vi "Double Click Action Data.vi"(7 "Row":i32, 8 "Action List":T2(array[cluster])=[{"Action Name"="Enable Motor", "JSON info"=[{"path"="Index", "data type"=enum."INT"}], "String Format"="%(Action Name) %(Index)"}, {"Action Name"="Disable Motor", "JSON info"=[{"path"="Index", "data type"=enum."INT"}], "String Format"="%(Action Name) %(Index)"}, {"Action Name"="Move Motor", "JSON info"=[{"path"="Index", "data type"=enum."INT"}, {"path"="Destination", "data type"=enum."DBL"}], "String Format"="%(Action Name) %(Index) to %(Destination)"}], 9 "Array of Data Types in":T1(array[cluster]), 10 "Array of Data Names&Defaults in":cluster{"Data Names&Defaults":string[][]}[](array[cluster]), 11 "MCListbox Ref":refnum<vi>) -> (1 "Array of Data Types out":T1(array[cluster]), 2 "Array of Data Names&Defaults out":cluster{"Data Names&Defaults":string[][]}[](array[cluster]))   [LabVIEW 2016, in "Hardware.lvlib" / "Motions.lvlib" / "Motions.lvclass"]
uses:
  <userlib>/Common Components/Hardware/Abstract System/Motions/Motions/Motions.lvclass
  <userlib>/TSPopup/TSPopup.lvlib
panel:
  in  "Motor Labels":string[](array[string])
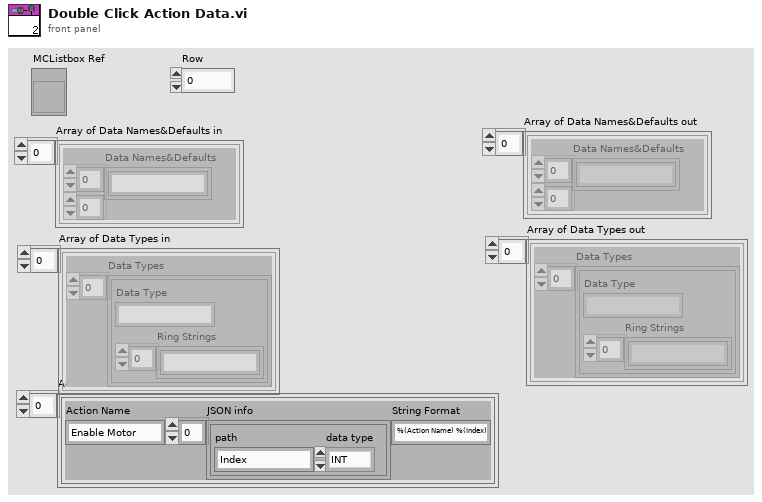
[diagram p1: front panel]
types:
  T1 = cluster{"Data Types":cluster{"Data Type":string, "Ring Strings":string[]}[]}[]
  T2 = cluster{"Action Name":string, "JSON info":cluster{"path":string, "data type":enum16{"INT", "DBL", "BOOL", "String"}}[], "String Format":string}[]
  T3 = cluster{"Data Type":string, "Captioned/Ring Strings":string[]}
  T4 = cluster{"path":string, "data type":enum16{"INT", "DBL", "BOOL", "String"}}[]
  T5 = cluster{"Data Types":cluster{"Data Type":string, "Ring Strings":string[]}[]}
  T6 = cluster{"Data Type":string, "Ring Strings":string[]}[]
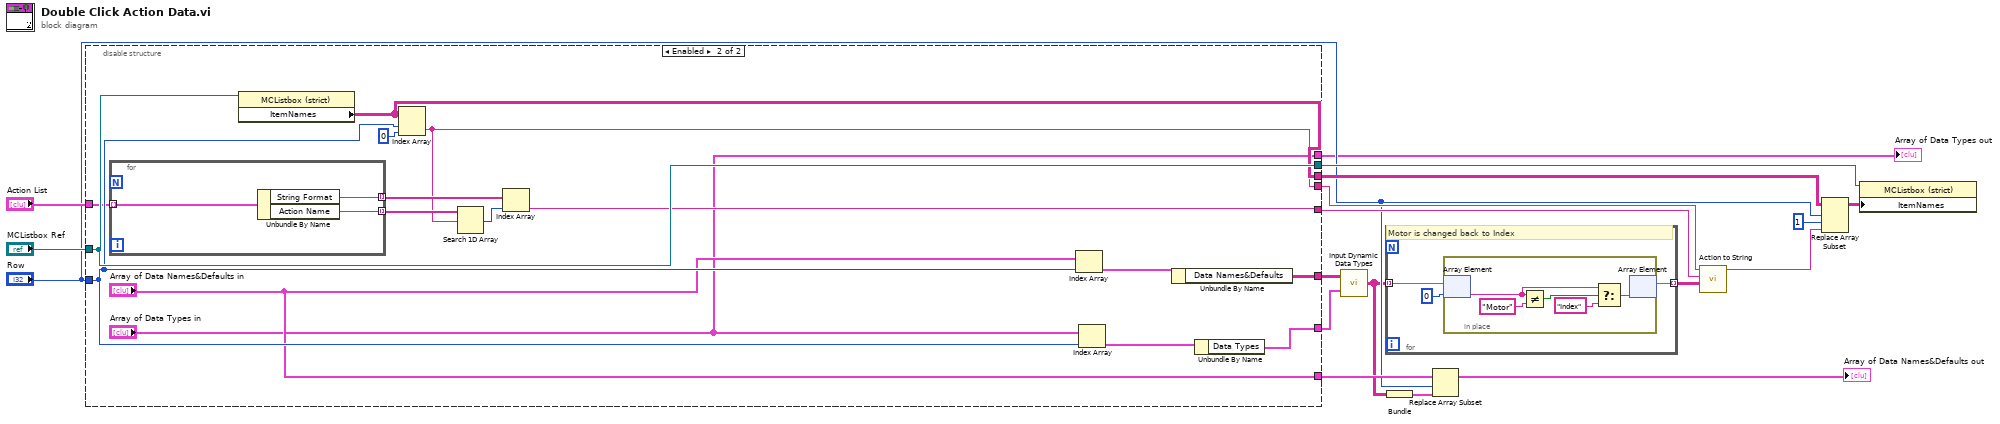
[diagram p0: block diagram]
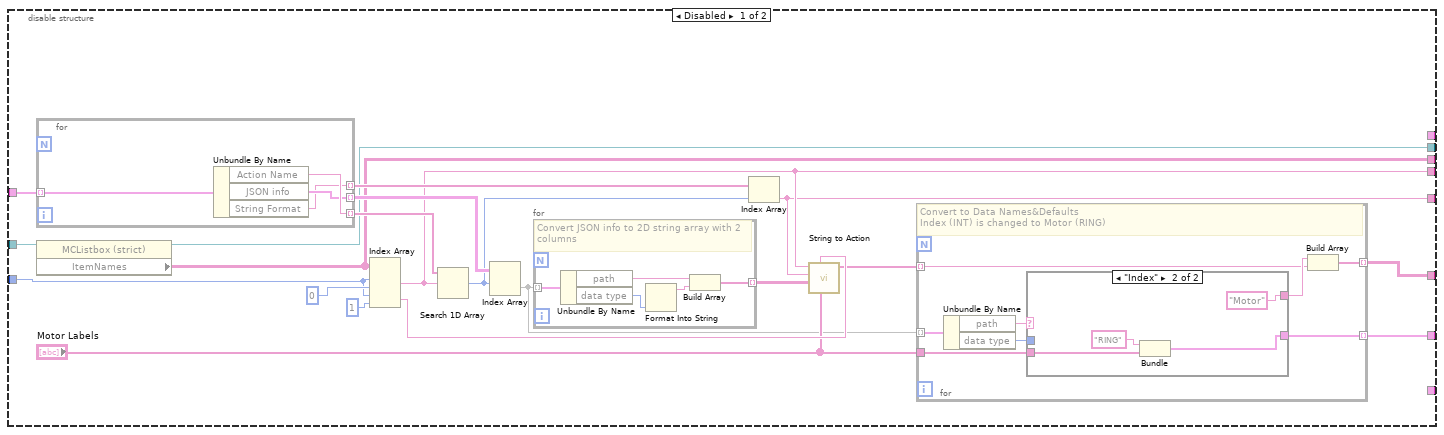
[diagram p2: hidden frame]
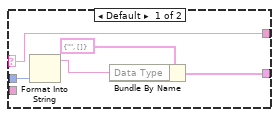
[diagram p3: hidden frame]
diagram:
  n1 = disable-structure shown="Enabled" {
    disable-tunnel: "MCListbox Ref" -> [w38 w78]
    disable-tunnel: "Action List" -> [w37 w74]
    disable-tunnel: [w33 w66] -> w16
    disable-tunnel: [w32 w65] -> w15
    disable-tunnel: [w29 w78] -> w14
    disable-tunnel: [w28 w77] -> w13
    disable-tunnel: "Row" -> [w27 w76]
    disable-tunnel: [w24 w71] -> w8
    disable-tunnel: [w23 w69] -> w7
    disable-tunnel: [_ "Array of Data Names&Defaults in"] -> w6
    disable-tunnel: [_ "Array of Data Types in"] -> w2
    frame Disabled {
      n2 = for {
        tunnel: w37 -> [w64] mode=indexing
        tunnel: [w63] -> w36 mode=indexing
        tunnel: [w62] -> w35 mode=indexing
        tunnel: [w61] -> w34 mode=indexing
        n3 = Unbundle By Name(w64) -> ("Action Name"=w63:string, "JSON info"=w62:T4, "String Format"=w61:string)
      }
      n4 = property class="MCListbox (strict)"(reference=w38) -> (reference out=w29:refnum<vi>, "ItemNames"=w28:string[][])  [unwired: 1 in, 1 out]
      n5 = Index Array(array=w28, index (row) #1=w27, index (col) #1=0 ("disabled index (col)"), index (row) #2=w27, index (col) #2=1 ("disabled index (col)")) -> (element #1=w24:string, element #2=w25:string)
      n6 = Search 1D Array(1D array=w36, element=w24) -> (index of element=w30:i32)  [unwired: 1 in]
      n7 = Index Array(array=w35, index (row)=w30) -> (element=w20:T4)  [unwired: 1 in]
      n8 = for {
        tunnel: w20 -> [w43] mode=indexing
        tunnel: [w39] -> w19 mode=indexing
        # "Convert JSON info to 2D string array with 2 columns"
        n9 = Unbundle By Name(w43) -> ("path"=w40:string, "data type"=w42:enum16{"INT", "DBL", "BOOL", "String"})
        n10 = Format Into String(w42) -> (resulting string=w41:string)  [unwired: 3 in, 1 out]
        n11 = Build Array(w40, w41) -> (w39:string[])
      }
      n12 = Index Array(array=w34, index=w30) -> (element=w23:string)
      n13 = call <userlib>:"String to Action.vi"("Motor Labels"="Motor Labels", "String"=w25, "Data Names&Types"=w19, "String Format"=w23, "Action Name"=w24) -> ("Data"=w21:string[])  [unwired: 5 in, 1 out]
      n14 = for {
        tunnel: w20 -> [w51] mode=indexing
        tunnel: [w45] -> w33 mode=indexing
        tunnel: "Motor Labels" -> [w49]
        tunnel: [w48] -> w32 mode=indexing
        tunnel: w21 -> [w44] mode=indexing
        # "Convert to Data Names&Defaults\nIndex (INT) is changed to Motor (RING)"
        n15 = Unbundle By Name(w51) -> ("path"=w50:string, "data type"=w47:enum16{"INT", "DBL", "BOOL", "String"})
        n16 = case shown="\"Index\"" w50 {
          selector: w50 -> [w52 _]
          tunnel: [w52 "Motor" ("element")] -> w46
          tunnel: w49 -> [_ w59]
          tunnel: [w53 w58] -> w48
          tunnel: w47 -> [w56 _]
          frame Default {
            n17 = Format Into String(w56) -> (resulting string=w54:string)  [unwired: 3 in, 1 out]
            n18 = Bundle By Name(cluster=T3 {"Data Type"="", "Captioned/Ring Strings"=[]}, "Data Type"=w54) -> (w53:T3)
          }
          frame "Index" {
            n19 = Bundle("RING", "Motor Labels"=w59) -> (w58:cluster{string, "Motor Labels":string[]})  [unwired: 1 in]
          }
        }
        n20 = Build Array(w46, w44) -> (w45:string[])
      }
    }
    frame Enabled {
      n21 = for {
        tunnel: w74 -> [w83] mode=indexing
        tunnel: [w82] -> w73 mode=indexing
        tunnel: [w81] -> w72 mode=indexing
        n22 = Unbundle By Name(w83) -> ("String Format"=w82:string, "Action Name"=w81:string)
      }
      n23 = property class="MCListbox (strict)"(reference=w78) -> ("ItemNames"=w77:string[][])  [unwired: 1 in, 2 out]
      n24 = Index Array(array=w77, index (row)=w76, index (col)=0 ("disabled index (col)")) -> (element=w71:string)
      n25 = Search 1D Array(1D array=w72, element=w71) -> (index of element=w70:i32)  [unwired: 1 in]
      n26 = Index Array(array=w73, index=w70) -> (element=w69:string)
      n27 = Index Array(array="Array of Data Names&Defaults in", index=w76) -> (element=w80:cluster{"Data Names&Defaults":string[][]})
      n28 = Index Array(array="Array of Data Types in", index=w76) -> (element=w79:T5)
      n29 = Unbundle By Name(w80) -> ("Data Names&Defaults"=w66:string[][])
      n30 = Unbundle By Name(w79) -> ("Data Types"=w65:T6)
    }
  }
  "Array of Data Types out" <- w2
  n31 = call <userlib>:"Input Dynamic Data Types.vi"("Data Types"=w15, "Data Names&Defaults"=w16) -> ("Data Names&Data"=w4:string[][])
  n32 = for {
    tunnel: w4 -> [w86] mode=indexing
    tunnel: [w84] -> w9 mode=indexing
    # "Motor is changed back to Index"
    n33 = in-place {
      n34 = in-place-array #1(w86, 0) -> (w89:string)
      n35 = Not Equal?(x=w89, y="Motor" ("element")) -> (x != y?=w90:bool)
      n36 = Select(t=w89, s=w90, f="Index" ("element")) -> (s? t:f=w87:string)
      n37 = in-place-array #1(w87) -> (w84:string[])  [unwired: 1 out]
    }
  }
  n38 = Bundle("Data Names&Data"=w4) -> (w1:cluster{"Data Names&Data":string[][]})  [unwired: 1 in]
  n39 = Replace Array Subset(array=w6, new element=w1, index="Row") -> (→"Array of Data Names&Defaults out":cluster{"Data Names&Defaults":string[][]}[])
  n40 = call <userlib>:"Action to String.vi"("Action Data"=w9, "String Format"=w7, "Action Name"=w8) -> ("String"=w11:string)  [unwired: 7 in, 1 out]
  n41 = Replace Array Subset(array=w13, new element=w11, index (row)="Row", index (col)=1 ("disabled index (col)")) -> (w10:string[][])
  n42 = property class="MCListbox (strict)"(reference=w14, "ItemNames"=w10) -> ()  [unwired: 1 in, 2 out]
